vi "XY Plot - Y Scale - Position - Left--Const.vi"() -> (3 "Y Scale.Position:Left":i32)   [LabVIEW 2017, in "DTacq Plot Display Library.lvlib"]
uses:
  DTacq Plot Display Library.lvlib
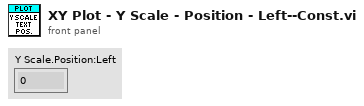
[diagram p1: front panel]
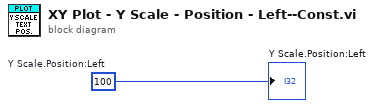
[diagram p0: block diagram]
diagram:
  w1 = 100  # Y Scale.Position:Left
  "Y Scale.Position:Left" <- w1
